vi "振动监测界面.vi"() -> ()   [LabVIEW 2016, in "环境动力监测库.lvlib"]
uses:
  <vilib>/ptbypt/NI_PtbyPt.lvlib
panel:
  out "振动监测":bool
  # "振动监测"
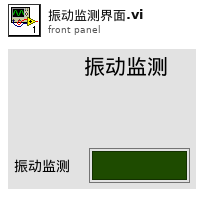
[diagram p1: front panel]
types:
  T1 = cluster{"漏水监测配置":cluster{"监测项描述:输出":string, "端口:":enum16{"AI0", "AI1", "AI2", "AI3", "AI4", "DI0", "DI1", "DI2", "DI3", "DI4", "DO0", "DO1", "DO2", "DO3", "DO4", "X0", "X1", "X2", "X3", "X4", "X5", "X6", "X7", "X8", "X9"}, "告警参数:":enum32{"禁用告警", "闭合告警", "断开告警"}, "传感器型号:":enum16{"PLC", "ZLAN"}}, "门禁开关监测配置":cluster{"监测项描述:输出":string, "端口:":enum16{"AI0", "AI1", "AI2", "AI3", "AI4", "DI0", "DI1", "DI2", "DI3", "DI4", "DO0", "DO1", "DO2", "DO3", "DO4", "X0", "X1", "X2", "X3", "X4", "X5", "X6", "X7", "X8", "X9"}, "告警参数:":enum32{"禁用告警", "闭合告警", "断开告警"}, "传感器型号:":enum16{"PLC", "ZLAN"}}, "温湿度监测配置":cluster{"监测项描述:输出":string, "端口:":enum16{"AI0", "AI1", "AI2", "AI3", "AI4", "DI0", "DI1", "DI2", "DI3", "DI4", "DO0", "DO1", "DO2", "DO3", "DO4", "X0", "X1", "X2", "X3", "X4", "X5", "X6", "X7", "X8", "X9"}, "告警参数:":enum32{"禁用告警", "闭合告警", "断开告警"}, "传感器型号:":enum16{"PLC", "ZLAN"}}, "烟雾监测配置":cluster{"监测项描述:输出":string, "端口:":enum16{"AI0", "AI1", "AI2", "AI3", "AI4", "DI0", "DI1", "DI2", "DI3", "DI4", "DO0", "DO1", "DO2", "DO3", "DO4", "X0", "X1", "X2", "X3", "X4", "X5", "X6", "X7", "X8", "X9"}, "告警参数:":enum32{"禁用告警", "闭合告警", "断开告警"}, "传感器型号:":enum16{"PLC", "ZLAN"}}, "冰箱监测配置":cluster{"监测项描述:输出":string, "端口:":enum16{"AI0", "AI1", "AI2", "AI3", "AI4", "DI0", "DI1", "DI2", "DI3", "DI4", "DO0", "DO1", "DO2", "DO3", "DO4", "X0", "X1", "X2", "X3", "X4", "X5", "X6", "X7", "X8", "X9"}, "告警参数:":enum32{"禁用告警", "闭合告警", "断开告警"}, "传感器型号:":enum16{"PLC", "ZLAN"}}, "排气扇监测配置":cluster{"监测项描述:输出":string, "端口:":enum16{"AI0", "AI1", "AI2", "AI3", "AI4", "DI0", "DI1", "DI2", "DI3", "DI4", "DO0", "DO1", "DO2", "DO3", "DO4", "X0", "X1", "X2", "X3", "X4", "X5", "X6", "X7", "X8", "X9"}, "告警参数:":enum32{"禁用告警", "闭合告警", "断开告警"}, "传感器型号:":enum16{"PLC", "ZLAN"}}}
  T2 = cluster{"监测项描述:输出":string, "端口:":enum16{"AI0", "AI1", "AI2", "AI3", "AI4", "DI0", "DI1", "DI2", "DI3", "DI4", "DO0", "DO1", "DO2", "DO3", "DO4", "X0", "X1", "X2", "X3", "X4", "X5", "X6", "X7", "X8", "X9"}, "告警参数:":enum32{"禁用告警", "闭合告警", "断开告警"}, "传感器型号:":enum16{"PLC", "ZLAN"}}
  T3 = enum16{"AI0", "AI1", "AI2", "AI3", "AI4", "DI0", "DI1", "DI2", "DI3", "DI4", "DO0", "DO1", "DO2", "DO3", "DO4", "X0", "X1", "X2", "X3", "X4", "X5", "X6", "X7", "X8", "X9"}
  T4 = cluster{"状态":cluster{"R0":i16, "R1":i16, "R2":i16, "R3":i16, "R4":i16, "R5":i16, "R6":i16, "R7":i16, "R8":i16, "R9":i16, "R10":i16, "R11":i16, "R12":i16, "R13":i16, "R14":i16, "R15":i16, "R16":i16, "R17":i16, "R18":i16, "R19":i16, "R20":i16, "R21":i16, "R22":i16, "R23":i16, "R24":i16, "R25":i16, "R26":i16, "R27":i16, "R28":i16, "R29":i16, "R30":i16, "R31":i16, "R32":i16, "R33":i16, "R34":i16, "R35":i16, "R36":i16, "R37":i16, "R38":i16, "R39":i16}, "输入状态":bool[], "输出状态":bool[], "参数设置":cluster{"R100":i16, "R101":i16, "R102":i16, "R103":i16, "R104":i16, "R105":i16, "R106":i16, "R107":i16, "R108":i16, "R109":i16, "R110":i16, "R111":i16, "R112":i16, "R113":i16, "R114":i16, "R115":i16, "R116":i16, "R117":i16, "R118":i16, "R119":i16, "R120":i16, "R121":i16, "R122":i16, "R123":i16}, "转换值":cluster{"AD0":sgl, "AD1":sgl, "AD2":sgl, "AD3":sgl, "AD4":sgl, "AD5":sgl}}
  T5 = cluster{"状态":cluster{"R0":i16, "R1":i16, "R2":i16, "R3":i16, "R4":i16, "R5":i16, "R6":i16, "R7":i16, "R8":i16, "R9":i16, "R10":i16, "R11":i16, "R12":i16, "R13":i16, "R14":i16, "R15":i16, "R16":i16, "R17":i16, "R18":i16, "R19":i16, "R20":i16, "R21":i16, "R22":i16, "R23":i16, "R24":i16, "R25":i16, "R26":i16, "R27":i16, "R28":i16, "R29":i16, "R30":i16, "R31":i16, "R32":i16, "R33":i16, "R34":i16, "R35":i16, "R36":i16, "R37":i16, "R38":i16, "R39":i16, "R40":i16, "R41":i16, "R42":i16, "R43":i16, "R44":i16, "R45":i16, "R46":i16, "R47":i16, "R48":i16, "R49":i16, "R50":i16, "R51":i16, "R52":i16, "R53":i16, "R54":i16, "R55":i16, "R56":i16, "R57":i16, "R58":i16, "R59":i16, "R60":i16, "R61":i16, "R62":i16, "R63":i16, "R64":i16, "R65":i16, "R66":i16, "R67":i16, "R68":i16, "R69":i16}, "输入状态":bool[], "输出状态":bool[], "报警簇":bool[], "参数设置":cluster{"R100":i16, "R101":i16, "R102":i16, "R103":i16, "R104":i16, "R105":i16, "R106":i16, "R107":i16, "R108":i16, "R109":i16, "R110":i16, "R111":i16, "R112":i16, "R113":i16, "R114":i16, "R115":i16, "R116":i16, "R117":i16, "R118":i16, "R119":i16, "R120":i16, "R121":i16, "R122":i16, "R123":i16, "R124":i16}, "转换值":cluster{"AD0":sgl, "AD1":sgl, "AD2":sgl, "AD3":sgl, "AD4":sgl, "AD5":sgl}, "看门狗启用":bool, "氨氮模块名称":string, "总磷模块名称":string}
  T6 = cluster{"环境变量":cluster{"蓄电池电压":dbl, "室温":dbl, "湿度":dbl, "水浸报警":bool, "烟雾报警":bool, "门禁1状态":bool, "门禁2状态":bool}, "ZLAN 6842 MB session":refnum<class "MB_Master.lvclass">, "DI":bool[], "DO":bool[], "AD当前转换值":cluster{"AD0":dbl, "AD1":dbl, "AD2":dbl, "AD3":dbl, "AD4":dbl, "AD5":dbl, "AD6":dbl, "AD7":dbl}}
  T7 = cluster{"漏水监测输出":bool, "门禁监测输出":bool, "温湿度监测输出":bool, "烟雾监测输出":bool, "空调监测输出":bool, "自动重合闸输出":bool, "红外入侵输出":bool, "振动输出":bool, "UPS输出":bool, "蓄电池输出":bool}
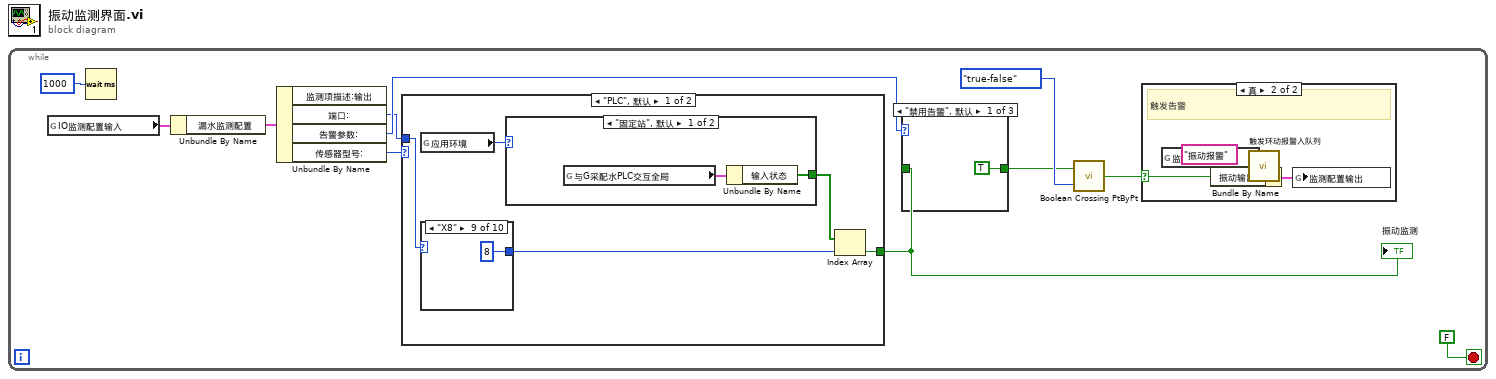
[diagram p0: block diagram]
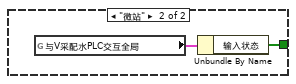
[diagram p2: hidden frame]
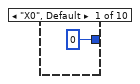
[diagram p3: hidden frame]
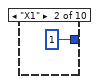
[diagram p4: hidden frame]
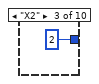
[diagram p5: hidden frame]
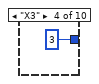
[diagram p6: hidden frame]
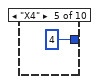
[diagram p7: hidden frame]
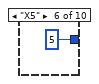
[diagram p8: hidden frame]
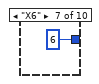
[diagram p9: hidden frame]
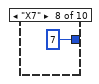
[diagram p10: hidden frame]
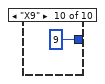
[diagram p11: hidden frame]
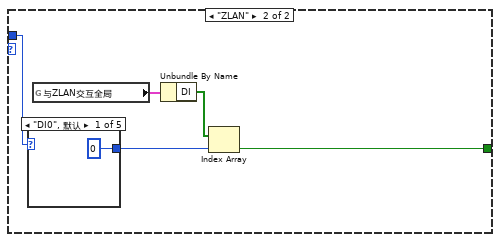
[diagram p12: hidden frame]
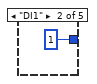
[diagram p13: hidden frame]
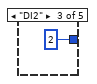
[diagram p14: hidden frame]
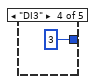
[diagram p15: hidden frame]
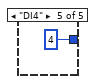
[diagram p16: hidden frame]
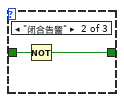
[diagram p18: hidden frame]
diagram:
  n1 = while {
    stop <- FALSE stop-if-true
    n2 = global read "断电保存全局变量.vi" "IO监测配置输入"() -> (w6:T1)
    n3 = Wait (ms)(milliseconds to wait=u32 1000 ("等待时间（毫秒）")) -> ()  [unwired: 1 out]
    n4 = Unbundle By Name(w6) -> ("漏水监测配置"=w11:T2)
    n5 = Unbundle By Name(w11) -> ("端口:"=w4:T3, "告警参数:"=w10:enum32{"禁用告警", "闭合告警", "断开告警"}, "传感器型号:"=w5:enum16{"PLC", "ZLAN"})  [unwired: 1 out]
    n6 = case shown="\"PLC\", 默认" w5 {
      tunnel: w4 -> [w16 w35]
      tunnel: [w14 w33] -> w3
      frame "PLC", Default {
        n7 = global read "外部交互全局变量.vi" "应用环境"() -> (w12:enum16{"固定站", "微站", "浮标", "浮船"})
        n8 = case shown="\"X8\"" w16 {
          tunnel: [0 ("索引") 1 ("索引") 2 ("索引") 3 ("索引") 4 ("索引") 5 ("索引") 6 ("索引") 7 ("索引") 8 ("索引") 9 ("索引")] -> w15
          frame "X0", Default {
          }
          frame "X1" {
          }
          frame "X2" {
          }
          frame "X3" {
          }
          frame "X4" {
          }
          frame "X5" {
          }
          frame "X6" {
          }
          frame "X7" {
          }
          frame "X8" {
          }
          frame "X9" {
          }
        }
        n9 = case shown="\"固定站\", 默认" w12 {
          tunnel: [w17 w19] -> w13
          frame "固定站", Default {
            n10 = global read "外部交互全局变量.vi" "与G采配水PLC交互全局"() -> (w18:T4)
            n11 = Unbundle By Name(w18) -> ("输入状态"=w17:bool[])
          }
          frame "微站" {
            n12 = global read "外部交互全局变量.vi" "与V采配水PLC交互全局"() -> (w20:T5)
            n13 = Unbundle By Name(w20) -> ("输入状态"=w19:bool[])
          }
        }
        n14 = Index Array(array=w13, index=w15) -> (element=w14:bool)
      }
      frame "ZLAN" {
        n15 = case shown="\"DI0\", 默认" w35 {
          tunnel: [0 ("索引") 1 ("索引") 2 ("索引") 3 ("索引") 4 ("索引")] -> w34
          frame "DI0", Default {
          }
          frame "DI1" {
          }
          frame "DI2" {
          }
          frame "DI3" {
          }
          frame "DI4" {
          }
        }
        n16 = global read "外部交互全局变量.vi" "与ZLAN交互全局"() -> (w32:T6)
        n17 = Unbundle By Name(w32) -> ("DI"=w31:bool[])
        n18 = Index Array(array=w31, index=w34) -> (element=w33:bool)
      }
    }
    "振动监测" <- w3
    n19 = case shown="\"禁用告警\", 默认" w10 {
      tunnel: w3 -> [_ w47 w48]
      tunnel: [TRUE ("漏水监测输出") w46 w48] -> w1
      frame "禁用告警", Default {
      }
      frame "闭合告警" {
        n20 = Not(x=w47) -> (.not. x?=w46:bool)
      }
      frame "断开告警" {
      }
    }
    n21 = call <vilib>:"Boolean Crossing PtByPt.vi"("direction"=enum16{"either", "false-true", "true-false"}."true-false", "input"=w1) -> ("crossing"=w2:bool)  [unwired: 1 in]
    n22 = case shown="真" w2 {
      selector: w2 -> [_ w41]
      frame False {
      }
      frame True {
        # "触发告警"
        n23 = global read "断电保存全局变量.vi" "监测配置输出"() -> (w42:T7)
        n24 = Bundle By Name(cluster=w42, "振动输出"=w41) -> (w43:T7)
        n25 = call "触发环动报警入队列.vi"("报警内容"="振动报警") -> ()  [unwired: 11 in]
        n26 = global write "断电保存全局变量.vi" "监测配置输出"(w43) -> ()
      }
    }
  }
